vi "odczyt.vi"(0 "refnum in":refnum<file>, 5 "error in":errorcluster) -> (6 "Thin":dbl, 8 "Thout":dbl, 10 "F1":dbl, 12 "Pnom":dbl, 14 "refnum out":refnum<file>, 19 "error out":errorcluster)   [LabVIEW 2023]
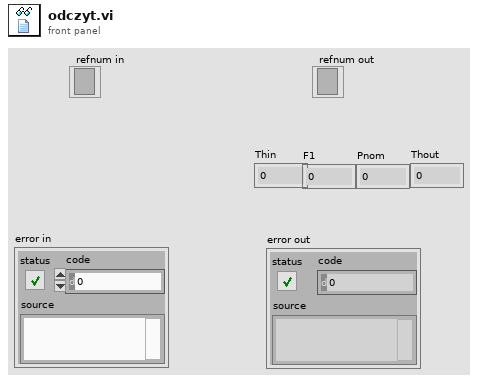
[diagram p1: front panel]
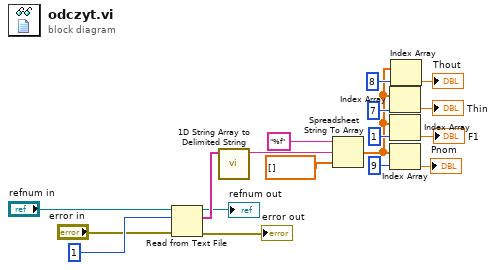
[diagram p0: block diagram]
diagram:
  n1 = Read from Text File(file (use dialog)="refnum in", count=1, error in="error in") -> (refnum out=→"refnum out":refnum<file>, text=w17:string[], error out=→"error out":errorcluster)  [unwired: 1 in, 1 out]
  n2 = call <vilib>:"1D String Array to Delimited String.vi"("string array"=w17) -> ("delimited string"=w16:string)  [unwired: 10 in]
  n3 = Spreadsheet String To Array(format string="%f", spreadsheet string=w16, array type (2D Dbl)=dbl[] [] ("array type (1D Dbl)")) -> (array=w1:dbl[])  [unwired: 1 in]
  n4 = Index Array(array=w1, index=7) -> (element=→"Thin":dbl)
  n5 = Index Array(array=w1, index=1) -> (element=→"F1":dbl)
  n6 = Index Array(array=w1, index=9) -> (element=→"Pnom":dbl)
  n7 = Index Array(array=w1, index=8) -> (element=→"Thout":dbl)
